vi "UI_Elmts_Reads[Labels]-Strg.vi"(8 "error in (no error)":errorcluster, 10 "Elmts Labels":string[](array[string]), 11 "UI_Actor in":refnum<class "UI_Actor.lvclass">) -> (0 "error out":errorcluster, 1 "Founds":bool[](array[boolean]), 2 "Values":string[](array[string]), 3 "UI_Actor out":refnum<class "UI_Actor.lvclass">)   [LabVIEW 2020, in "UI_Actor.lvlib" / "UI_Actor.lvclass"]
doc: "Accès à un élément par son label.\n<b> NEVER USE IN FOR LOOP </b> \nLa ref est stockée au premier appel en fgv.\nLe VI doit etre dédié à un unique élement."
uses:
  UI_Actor.lvclass
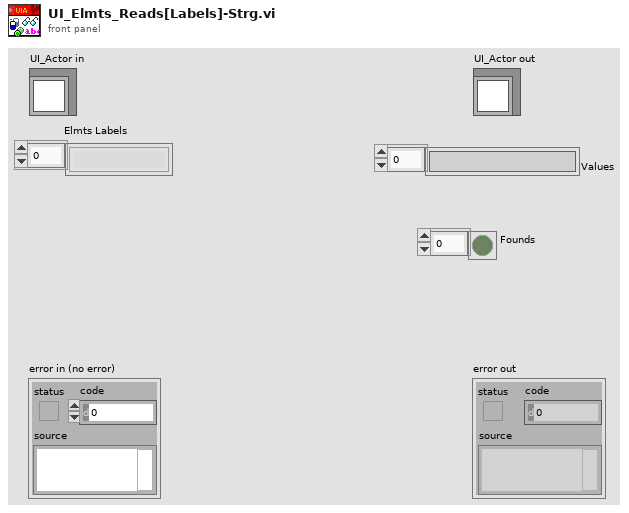
[diagram p1: front panel]
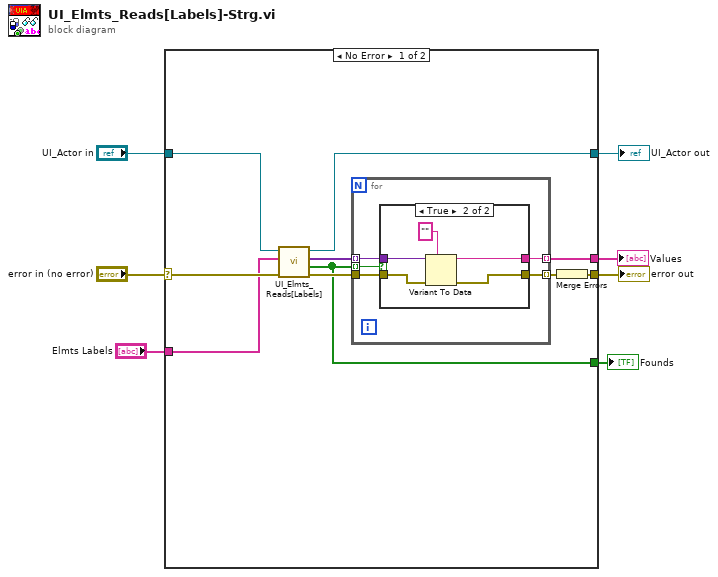
[diagram p0: block diagram]
diagram:
  n1 = case shown="No Error" "error in (no error)" {
    selector: "error in (no error)" -> [w14 w30]
    tunnel: [w8 w30] -> w6
    tunnel: [w12 w29] -> w4
    tunnel: "UI_Actor in" -> [w15 w29]
    tunnel: "Elmts Labels" -> [w11 _]
    tunnel: [w16 _] -> w2
    tunnel: [w10 _] -> w1
    frame No Error {
      n2 = call "UI_Elmts_Reads[Labels].vi"("error in (no error)"=w14, "Elmts Labels"=w11, "UI_Actor in"=w15) -> ("error out"=w13:errorcluster, "Founds"=w10:bool[], "Values"=w9:variant[], "UI_Actor out"=w12:refnum<class "UI_Actor.lvclass">)  [unwired: 5 in]
      n3 = for {
        tunnel: [w21] -> w16 mode=indexing
        tunnel: w10 -> [w19] mode=indexing
        tunnel: w9 -> [w18] mode=indexing
        tunnel: w13 -> [w20]
        tunnel: [w22] -> w17 mode=indexing
        n4 = case shown="True" w19 {
          tunnel: w18 -> [_ w28]
          tunnel: w20 -> [w23 w27]
          tunnel: [w23 w26] -> w22
          tunnel: [_ w24] -> w21
          frame False {
          }
          frame True {
            n5 = Variant To Data(error in=w27, type="", Variant=w28) -> (data=w24:string, error out=w26:errorcluster)
          }
        }
      }
      n6 = Merge Errors(w17) -> (w8:errorcluster)
    }
    frame Error {
    }
  }
  "error out" <- w6
  "UI_Actor out" <- w4
  "Values" <- w2
  "Founds" <- w1
